vi "beginFirstKick.vi"(8 "error in (no error)":errorcluster, 9 "Robot":refnum<class "Robot.lvclass">, 10 "Game":refnum<class "Game.lvclass">, 11 "WaitBallTrajSkill in":refnum<class "WaitBallTrajSkill.lvclass">) -> (0 "error out":errorcluster, 2 "Boolean":bool, 3 "WaitBallTrajSkill out":refnum<class "WaitBallTrajSkill.lvclass">)   [LabVIEW 2023, in "WaitBallTrajSkill.lvclass"]
uses:
  WaitBallTrajSkill.lvclass
  Game_class/Game.lvclass
  Robot_class/Robot.lvclass
  Game_class/Game.lvclass/Game.ctl
  Robot_class/Robot.lvclass/Robot.ctl
  NewSTP/Evaluators/PrimaryAttackerShot_class/PrimaryAttackerShot.lvclass
  Robot_class/Read role.vi
  Game_class/Read Utilities.lvclass.vi
  Game_class/Read BallRef.vi
  Game_class/Read KeeperTeam.vi
  Game_class/Read NewParameters.vi
  Game_class/Read FieldRef.vi
  Utilities_class/Utilities.lvclass
  Ball_class/Ball.lvclass
  Ally_class/Ally.lvclass
  Utilities_class/Style.ctl
  Field_class/Field.lvclass
  Zone_class/Zone.lvclass
  Team_class/KeeperPlay.ctl
panel:
  out "appended array":bool[](array[boolean])
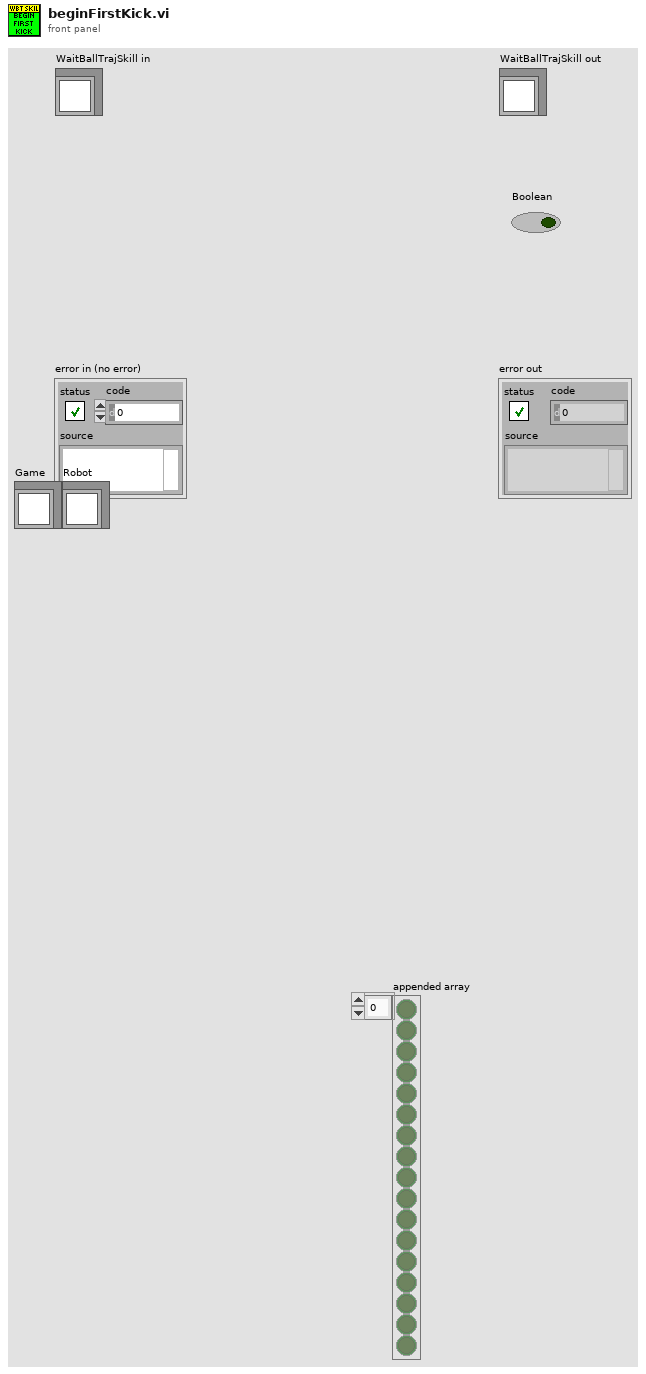
[diagram p1: front panel]
types:
  T1 = typedef "NewParameters.ctl" = cluster{"PenaltyDistance":dbl, "DistanceAttackerToBackBall":dbl, "Division":enum16{"Div B", "Div A"}, "DistanceToAvoidyEnemyRobot":dbl, "BallPlacementDistance":dbl, "DisatanceBehindBallToStealBall":dbl, "MaxDistanceToPositionKickoff":dbl, "BlockEnemyTarget":bool, "MaxStopVAng":dbl, "DistanceMarkerToEnemy":dbl, "IgnoreDribblerContact":bool, "DistanceToBeginEnemyPosession":dbl, "GoToBallWhenEnemyNotMoving":bool, "EnemyDistanceToReduceVelocity":dbl, "TurnOnEnemyDistanceToReduceVelocity":bool, "EnemyDistanceToShootOutBall":dbl, "DefenseKickBall":bool, "MoreKickToGoal? (0-0.3)":dbl, "ChipKickInEnemyField":bool, "ShootOutRobotId":dbl, "FieldLenghtDenominatorInShootOut":dbl, "AdjustPositionInBallPlacement":bool, "PowerGodPass":dbl, "VelocityAbortEnemyPos":dbl, "MaxDistToBeginPass":dbl, "MinDistToBeginPass":dbl, "VelocityInDirects":dbl, "BadDribblerIDs":i32[], "NewKickToDistanceAroundBall":dbl, "PowerAvoidColisionMarker":dbl, "DistanceToAvoidColisionMarker":dbl, "AvoidBallKick":dbl, "DistanceTryKick":dbl, "SuicideKickDIstance":dbl, "FirstKickAtck":bool, "AdjustFirstKickDistance":dbl, "FirstKickDefense":bool, "AvoidAimLessKick":dbl, "DistanceToAvoidyEnemyShootRobot ":dbl, "NumberOfMarkers":dbl, "PotField":bool, "PIDLateral":bool, "MinDistanceFirstKickX":dbl, "MinDistanceFirstKickY":dbl, "FractionOfDistToTouchGround\nAfterChipKick":dbl, "FractionOfKickxWhen\nComposedWithKickz":dbl, "Style":T2, "MoveInTurnState":bool, "DistFromEnemyToConsider\nMoveInTurnState":dbl, "CascadePID":bool, "TurnAroundParameters":cluster{"Radius":dbl, "Multiplier":dbl, "ChordAngle":dbl}, "SafeDriveVel":dbl, "DistanceToGoToBackBall":dbl, "minDistanceToNotFinishEnemyPossession":dbl, "Probability to kick direct penalty (0 - 1)":dbl}
  T2 = typedef "Style.ctl" = enum16{"Insanity", "Offensive", "Defensive"}
  T3 = typedef "STPParameters.ctl" = cluster{"Skills":T4, "TestSkill":T6, "Events":cluster{"distanceToBallPossession":dbl, "timeForPossessionThreshold":dbl}, "Criteria":cluster{"OpenAngleToGoal":cluster{"minAngle":dbl, "maxAngle":dbl, "minEvaluation":dbl}, "PassDistance":cluster{"maxDistance":dbl, "minDistance":dbl}, "ShotInterception":cluster{"shotSpeed":dbl, "minEnemySpeed":dbl, "minEvaluation":dbl, "maxEnemySpeed":dbl}, "OneTouchShot":cluster{"MaxAngle":dbl, "minEvaluation":dbl}, "PassInterception":cluster{"minEnemySpeed":dbl, "maxEnemySpeed":dbl, "chipPassDistance":dbl, "chipPassEval":dbl, "minEvaluation":dbl}}, "minPassSpeed":dbl, "maxPassSpeed":dbl, "AllyTeamIds":T7[], "ReceiverSpeed":dbl, "minEvaluationToShoot":dbl, "maxDefendersNumber":u8}
  T4 = typedef "Skills.ctl" = cluster{"CirculateBall":T5, "ProtectBall":cluster{"DistanceFromBall":dbl}}
  T5 = typedef "CIrculateSkillParameters.ctl" = cluster{"rotationAngle":dbl, "velocityFactor":dbl, "OrientationFactor":dbl}
  T6 = typedef "TestSkills.ctl" = enum16{"AlignSkill", "PassSkill", "CirculateBall", "OneTouchShotSkill", "KickToSkill_v2", "ShootSkill", "InterceptBall", "Exit", "GoToSkill_v2"}
  T7 = typedef "AllyTeam.ctl" = enum16{"Keeper", "Defender", "Attacker"}
  T8 = typedef "KeeperPlay.ctl" = enum16{"SimpleBallPlacementAlly", "BallPlacementAlly", "BallPlacementEnemy", "ZigZag", "Goto", "NormalGame", "KeeperPlay", "Halt", "Timeout", "PenaltyEnemy", "TestPlay"}
  T9 = typedef "roles.ctl" = enum16{"SimpleBallPlacement", "BallPlacementAllyPasser", "BallPlacementAllyReceiver", "BallPlacementEnemy", "5Robots5th", "PassBestReceiver", "5Robots4th", "5Robots3rd", "5Robots2nd", "5Robots1st", "PassBestRobot", "WaitPass", "ABCThirdKicker", "ABCFirstKicker", "ABCSecondKicker", "Tabler", "TableFinalizer", "PrepareRollToPassRoller", "PrepareRollToPassReceiver", "SimplePassRoll", "SimplePassRollReceiver", "PenaltyDefense", "PreparePassReceiver 2", "PreparePassReceiver 1", "PassObserver", "Timeout", "Goto", "ZigZag", "None", "BallOutOfField", "DefenderArea", "Duelist", "AttackerStop", "FollowAttacker", "KeeperRole", "KickPenalty", "AttackerAimGoal", "AttackerBlock", "Marker", "Halt", "Shoot", "PassKicker", "PassReceiver", "TestRole", "PenaltyAttacker", "PrimaryAttackerRole", "SupportAttackerRole"}
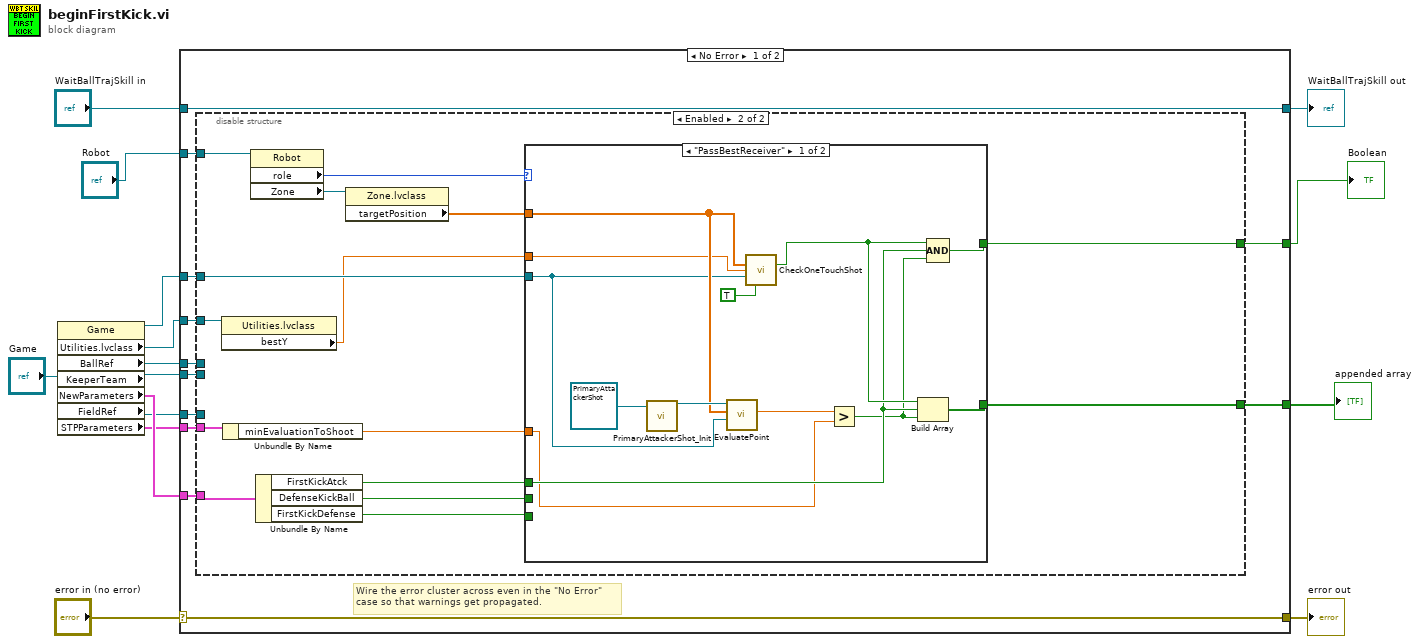
[diagram p0: block diagram]
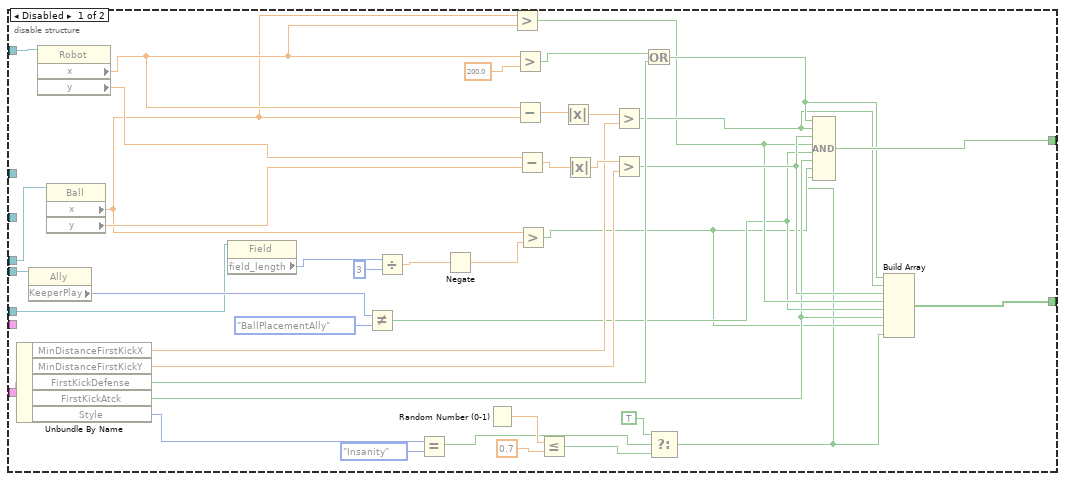
[diagram p2: hidden frame]
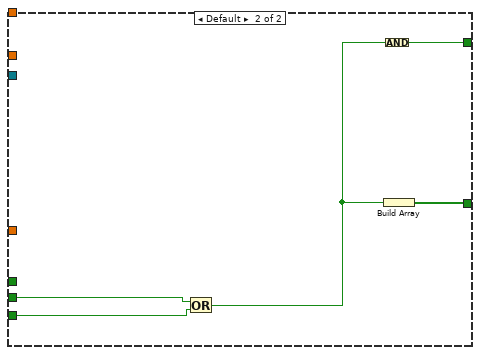
[diagram p3: hidden frame]
diagram:
  n1 = property class="Game"(reference="Game") -> (reference out=w4:refnum<class "Game.lvclass">, "Utilities.lvclass"=w1:refnum<class "Utilities.lvclass">, "BallRef"=w9:refnum<class "Ball.lvclass">, "KeeperTeam"=w10:refnum<class "Ally.lvclass">, "NewParameters"=w7:T1, "FieldRef"=w5:refnum<class "Field.lvclass">, "STPParameters"=w2:T3)  [unwired: 1 in, 1 out]
  n2 = case shown="No Error" "error in (no error)" {
    selector: "error in (no error)" -> [w26 w103]
    tunnel: [w26 w103] -> w14
    tunnel: [w27 w102] -> w12
    tunnel: "WaitBallTrajSkill in" -> [w27 w102]
    tunnel: w10 -> [w25 _]
    tunnel: w9 -> [w24 _]
    tunnel: "Robot" -> [w23 _]
    tunnel: w7 -> [w22 _]
    tunnel: [w21 _] -> w3
    tunnel: [w20 _] -> w6
    tunnel: w5 -> [w19 _]
    tunnel: w4 -> [w18 _]
    tunnel: w2 -> [w17 _]
    tunnel: w1 -> [w16 _]
    frame No Error {
      # "Wire the error cluster across even in the \"No Error\"\ncase so that warnings get propagated."
      n3 = disable-structure shown="Enabled" {
        disable-tunnel: w25 -> [w67 _]
        disable-tunnel: w24 -> [w65 _]
        disable-tunnel: w23 -> [w64 w83]
        disable-tunnel: w22 -> [w57 w81]
        disable-tunnel: [w53 w78] -> w21
        disable-tunnel: [w43 w79] -> w20
        disable-tunnel: w19 -> [w41 _]
        disable-tunnel: w18 -> [_ w77]
        disable-tunnel: w17 -> [_ w72]
        disable-tunnel: w16 -> [_ w70]
        frame Disabled {
          n4 = Unbundle By Name(w57) -> ("MinDistanceFirstKickX"=w55:dbl, "MinDistanceFirstKickY"=w54:dbl, "FirstKickDefense"=w56:bool, "FirstKickAtck"=w44:bool, "Style"=w34:T2)
          n5 = property class="Ally"(reference=w67) -> ("KeeperPlay"=w66:T8)  [unwired: 1 in, 2 out]
          n6 = property class="Robot"(reference=w64) -> ("x"=w52:dbl, "y"=w50:dbl)  [unwired: 1 in, 2 out]
          n7 = property class="Ball"(reference=w65) -> ("x"=w42:dbl, "y"=w51:dbl)  [unwired: 1 in, 2 out]
          n8 = property class="Field"(reference=w41) -> ("field_length"=w40:i32)  [unwired: 1 in, 2 out]
          n9 = Not Equal?(x=w66, y=KeeperPlay."BallPlacementAlly") -> (x != y?=w45:bool)
          n10 = Divide(x=w40, y=3) -> (x/y=w38:dbl)
          n11 = Equal?(x=w34, y=Style."Insanity") -> (x = y?=w31:bool)
          n12 = Negate(x=w38) -> (-x=w37:dbl)
          n13 = Random Number (0-1)() -> (number: 0 to 1=w36:dbl)
          n14 = Greater?(x=w42, y=w52) -> (0:w46:bool)
          n15 = Greater?(x=w52, y=200.0) -> (0:w58:bool)
          n16 = Subtract(x=w52, y=w42) -> (x-y=w62:dbl)
          n17 = Subtract(x=w50, y=w51) -> (x-y=w61:dbl)
          n18 = Greater?(x=w42, y=w37) -> (0:w29:bool)
          n19 = Less Or Equal?(x=w36, y=0.7) -> (x <= y?=w32:bool)
          n20 = Absolute Value(x=w62) -> (abs(x)=w60:dbl)
          n21 = Absolute Value(x=w61) -> (abs(x)=w59:dbl)
          n22 = Greater?(x=w60, y=w55) -> (0:w48:bool)
          n23 = Greater?(x=w59, y=w54) -> (0:w47:bool)
          n24 = Or(x=w58, y=w56) -> (x .or. y?=w49:bool)
          n25 = Select(t=TRUE, s=w31, f=w32) -> (s? t:f=w28:bool)
          n26 = Compound Arithmetic op=AND(w49, w48, w47, w46, w45, w44, w29, w28) -> (w53:bool)
          n27 = Build Array(w49, w48, w47, w46, w45, w44, w29, w28) -> (w43:bool[])
        }
        frame Enabled {
          n28 = property class="Utilities.lvclass"(reference=w70) -> ("bestY"=w69:dbl)  [unwired: 1 in, 2 out]
          n29 = Unbundle By Name(w72) -> ("minEvaluationToShoot"=w71:dbl)
          n30 = property class="Robot"(reference=w83) -> ("role"=w82:T9, "Zone"=w74:refnum<class "Zone.lvclass">)  [unwired: 1 in, 2 out]
          n31 = Unbundle By Name(w81) -> ("FirstKickAtck"=w75:bool, "DefenseKickBall"=w80:bool, "FirstKickDefense"=w76:bool)
          n32 = property class="Zone.lvclass"(reference=w74) -> ("targetPosition"=w73:dbl[])  [unwired: 1 in, 2 out]
          n33 = case shown="\"PassBestReceiver\"" w82 {
            tunnel: w80 -> [_ w99]
            tunnel: [w94 w101] -> w79
            tunnel: [w96 w100] -> w78
            tunnel: w77 -> [w84 _]
            tunnel: w73 -> [w90 _]
            tunnel: w76 -> [_ w98]
            tunnel: w75 -> [w93 _]
            tunnel: w71 -> [w87 _]
            tunnel: w69 -> [w86 _]
            frame "PassBestReceiver" {
              n34 = call "PrimaryAttackerShot_Init.vi"("object in"=refnum<class "PrimaryAttackerShot.lvclass"> refnum ("PrimaryAttackerShot")) -> ("object out"=w91:refnum<class "PrimaryAttackerShot.lvclass">)  [unwired: 17 in, 1 out]
              n35 = call-dynamic "EvaluatePoint.vi"("Game"=w84, "Point"=w90, "Evaluator in"=w91) -> ("Evaluation"=w89:dbl)  [unwired: 6 in, 2 out]
              n36 = call "CheckOneTouchShot.vi"("Point"=w90, "Best y"=w86, "Game"=w84, "Ally?"=TRUE) -> ("OneTouch"=w95:bool)  [unwired: 8 in, 3 out]
              n37 = Greater?(x=w89, y=w87) -> (0:w88:bool)
              n38 = Build Array(w95, w93, w88) -> (w94:bool[])
              n39 = Compound Arithmetic op=AND(w95, w93, w88) -> (w96:bool)
            }
            frame Default {
              n40 = Or(x=w99, y=w98) -> (x .or. y?=w97:bool)
              n41 = Build Array(w97) -> (w101:bool[])
              n42 = Compound Arithmetic op=AND(w97) -> (w100:bool)
            }
          }
        }
      }
    }
    frame Error {
    }
  }
  "error out" <- w14
  "WaitBallTrajSkill out" <- w12
  "Boolean" <- w3
  "appended array" <- w6
